vi "matrix conversion.vi"(10 "File Path":path=path "C:/Users/Green Beret/Documents/Visual Studio 2012/Projects/LightPipes/LightPipes/lp12src/LabView/images/target_retrieved_phase.pgm", 11 "number of rows (all:-1)":i32=-1) -> (3 "all rows":dbl[][](array[numeric]) format="%0.3f")   [LabVIEW 2012, in "LightPipes.lvlib"]
uses:
  LightPipes.lvlib
  <vilib>/Utility/file.llb/Read From Spreadsheet File (DBL).vi
panel:
  out "Intensity Graph":dbl[][](graph)
  in  "delimiter (\\t)":string=" "
  in  "max characters/row  (no limit:0)":i32
  out "EOF?":bool
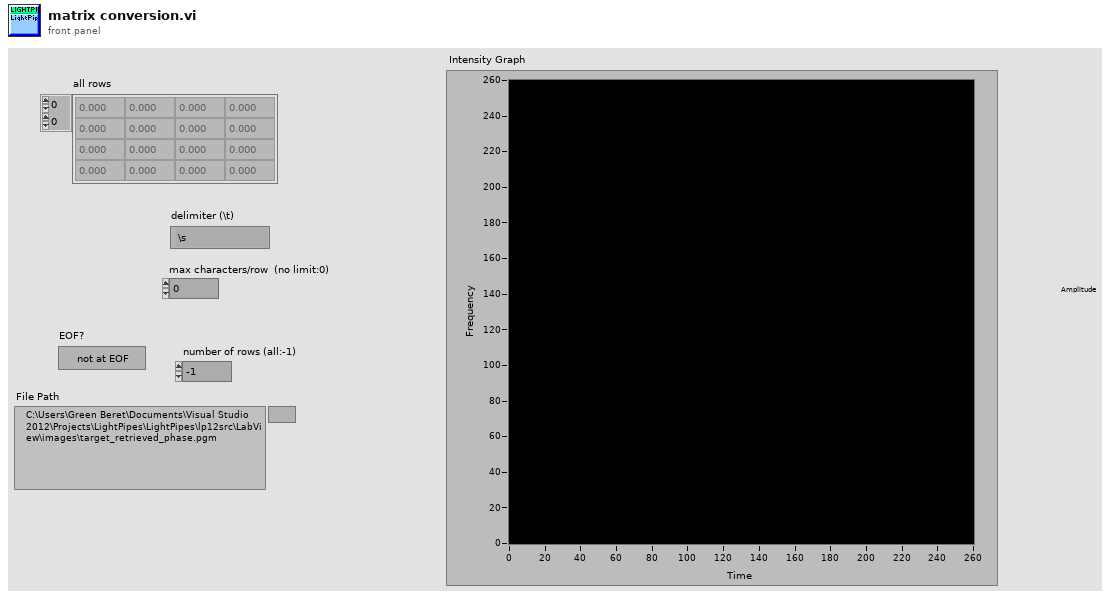
[diagram p1: front panel]
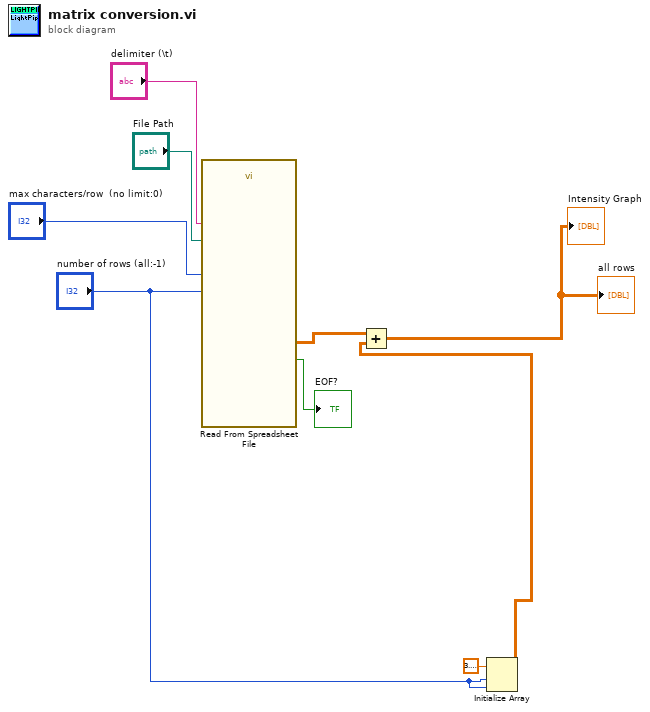
[diagram p0: block diagram]
diagram:
  n1 = call-poly <vilib>:"Read From Spreadsheet File.vi"("delimiter (\\t)"="delimiter (\\t)", "max characters/row  (no limit:0)"="max characters/row  (no limit:0)", "number of rows (all:-1)"="number of rows (all:-1)", "file path (dialog if empty)"="File Path") -> ("EOF?"=→"EOF?":bool, "all rows"=w5:dbl[][])  [unwired: 3 in, 3 out]
  n2 = Initialize Array(3.141592653589793, "number of rows (all:-1)", "number of rows (all:-1)") -> (w2:dbl[][])
  n3 = Add ("Add.vi")(x=w5, y=w2) -> (x+y=→"all rows" →"Intensity Graph":dbl[][])
